vi "CarouselInitializationChecklist.vi"(11 "Startup Checklist In":T1) -> (3 "Startup Checklist Out":T1)   [LabVIEW 2013]
uses:
  OpenCarouselInitializationChecklist.ctl
panel:
  in  "Stop":bool
  in  "Check All Btn":bool
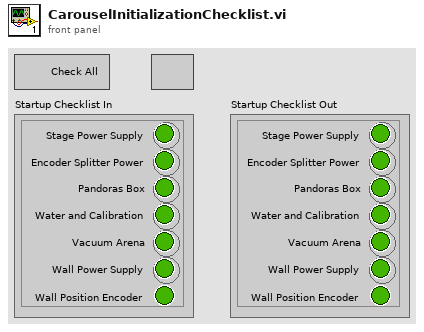
[diagram p1: front panel]
types:
  T1 = typedef "OpenCarouselInitializationChecklist.ctl" = cluster{"Encoder Splitter Power":bool, "Pandoras Box":bool, "Water and Calibration":bool, "Vacuum Arena":bool, "Wall Power Supply":bool, "Wall Position Encoder":bool, "Stage Power Supply":bool}
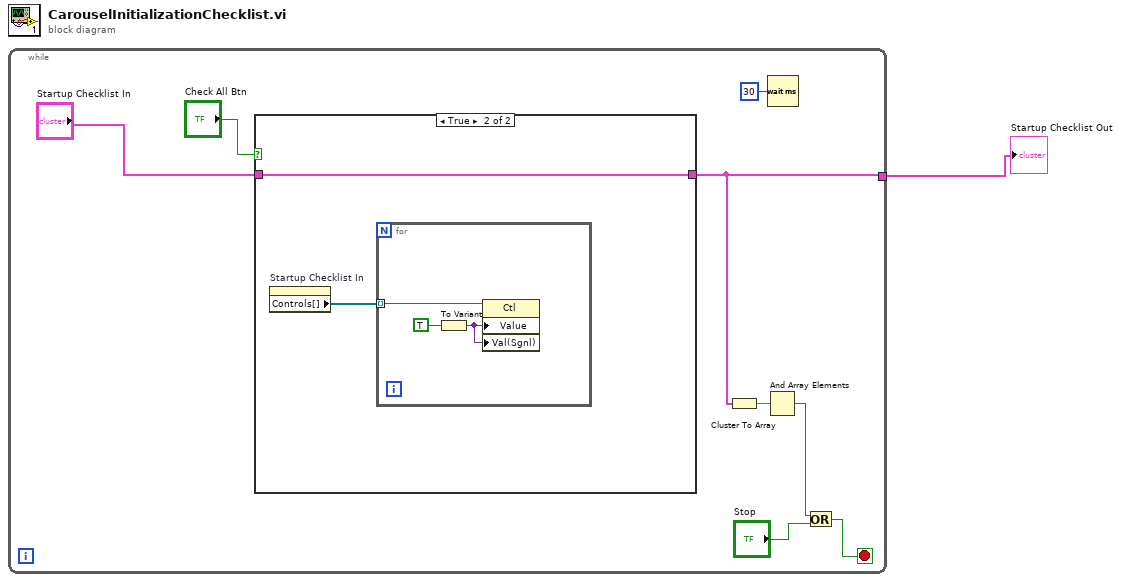
[diagram p0: block diagram]
diagram:
  n1 = while {
    tunnel: [w3] -> w1
    stop <- w7 stop-if-true
    n2 = case shown="True" "Check All Btn" {
      tunnel: "Startup Checklist In" -> [w10 w12]
      tunnel: [w10 w12] -> w3
      frame False {
      }
      frame True {
        n3 = property on="Startup Checklist In" class="Clust (strict)"() -> ("Controls[]"=w11:refnum<vi>[])  [unwired: 2 in, 2 out]
        n4 = for {
          tunnel: w11 -> [w14] mode=indexing
          n5 = To Variant(anything=TRUE) -> (Variant=w13:variant)
          n6 = property class="Ctl"(reference=w14, "Value"=w13, "Val(Sgnl)"=w13) -> ()  [unwired: 1 in, 2 out]
        }
      }
    }
    n7 = Cluster To Array(cluster=w3) -> (array=w4:bool[])
    n8 = And Array Elements(Boolean array=w4) -> (logical AND=w6:bool)
    n9 = Wait (ms)(milliseconds to wait=u32 30) -> ()  [unwired: 1 out]
    n10 = Or(x=w6, y="Stop") -> (x .or. y?=w7:bool)
  }
  "Startup Checklist Out" <- w1
